vi "Pre Launch Init.vi"(11 "Create Test Channel View in":refnum<class "Create Test Channel View.lvclass">) -> (0 "error out":errorcluster, 3 "Create Test Channel View out":refnum<class "Create Test Channel View.lvclass">)   [LabVIEW 2013, in "Create Test Channel View.lvlib" / "Create Test Channel View.lvclass"]
doc: "(<B>Filename</B>: Actor Framework.lvlib:Actor.lvclass:Pre Launch Init.vi)\n\nDefines behavior that occurs after the Launch Actor method is invoked but before the actor's Actor Core method begins running.\n\nThe Pre Launch Init method is guaranteed to finish before the Launch Actor method returns to its caller and before the actor itself receives any messages. Any references that the Pre Launch Init method obtains are guaranteed to have the same lifetime as the actor itself. Any errors that the Pre Launch Init method returns will abort the launch.\n\nBy default, this method does nothing. A descendant class may override it to define behavior."
uses:
  Create Test Channel View.lvclass
  Create Test Channel View.lvclass/Create Test Channel View.ctl
  <vilib>/ActorFrameworkMVC/View Actor/View Actor.lvclass
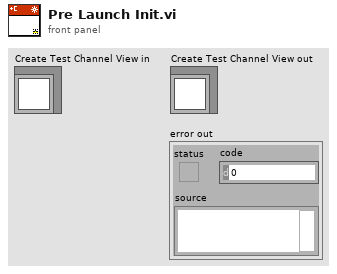
[diagram p1: front panel]
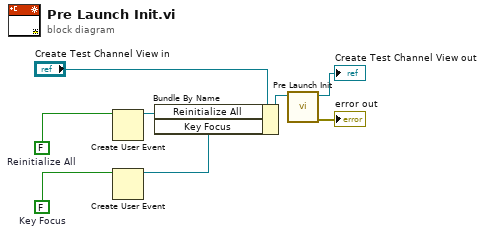
[diagram p0: block diagram]
diagram:
  w5 = FALSE  # Key Focus
  w6 = FALSE  # Reinitialize All
  n1 = Create User Event(user event datatype=w6) -> (user event=w4:refnum<user-event>)  [unwired: 1 in, 1 out]
  n2 = Create User Event(user event datatype=w5) -> (user event=w3:refnum<user-event>)  [unwired: 1 in, 1 out]
  n3 = Bundle By Name(cluster="Create Test Channel View in", "Reinitialize All"=w4, "Key Focus"=w3) -> (w1:refnum<class "Create Test Channel View.lvclass">)
  n4 = call-parent "Pre Launch Init.vi"("Actor in"=w1) -> ("error out"=→"error out":errorcluster, "Actor out"=→"Create Test Channel View out":refnum<class "Create Test Channel View.lvclass">)  [unwired: 9 in]
